vi "FTW-ActorRef-Close.vi"(0 "FTW Actor Reference":refnum<class "FTW-ActorReference.lvclass">, 11 "error in":errorcluster) -> (15 "error out":errorcluster)   [LabVIEW 2014, in "FTW-ActorReference.lvclass"]
uses:
  FTW-ActorReference.lvclass
panel:
  # "Inputs"
  # "Outputs"
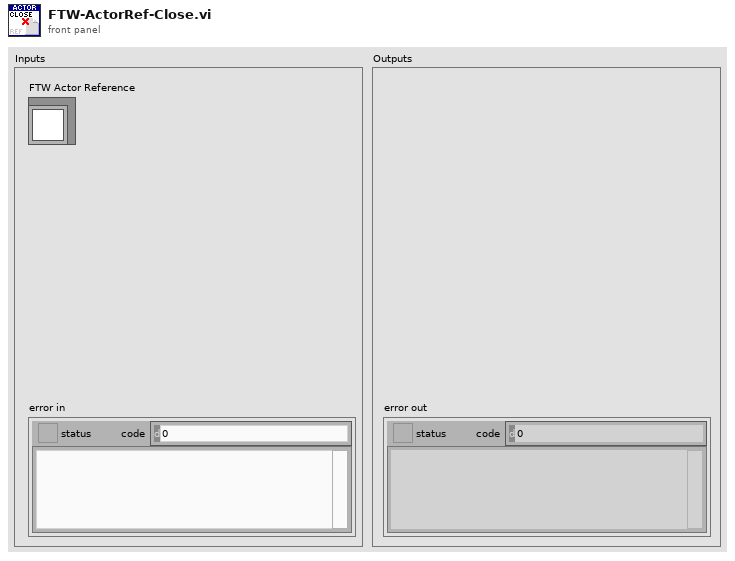
[diagram p1: front panel]
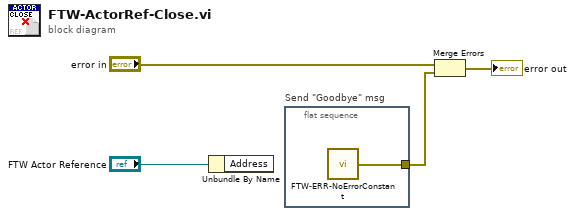
[diagram p0: block diagram]
diagram:
  n1 = Unbundle By Name("FTW Actor Reference") -> ()  [unwired: 1 out]
  n2 = flat-sequence "Send \"Goodbye\" msg" {
    tunnel: [w5] -> w1
    frame #0 {
      n3 = call "FTW-ERR-NoErrorConstant.vi"() -> ("no error"=w5:errorcluster)
    }
  }
  n4 = Merge Errors("error in", w1) -> (→"error out":errorcluster)
